vi "AB_820_850_Project_Build_Info.vi"(7 "action":T2, 8 "error in (no error)":errorcluster, 9 "buildType":T1, 10 "buildInfo in":T3, 11 "Object In":T4) -> (0 "error out":errorcluster, 2 "buildInfo out":T3, 3 "Object Out":T4)   [LabVIEW 2020]
uses:
  <resource>/Framework/Providers/API/ItemRef.ctl
  <vilib>/AppBuilder/RW_Project/AB_RW_Project_PropBag_Action.ctl
  <vilib>/AppBuilder/AB_BuildType.ctl
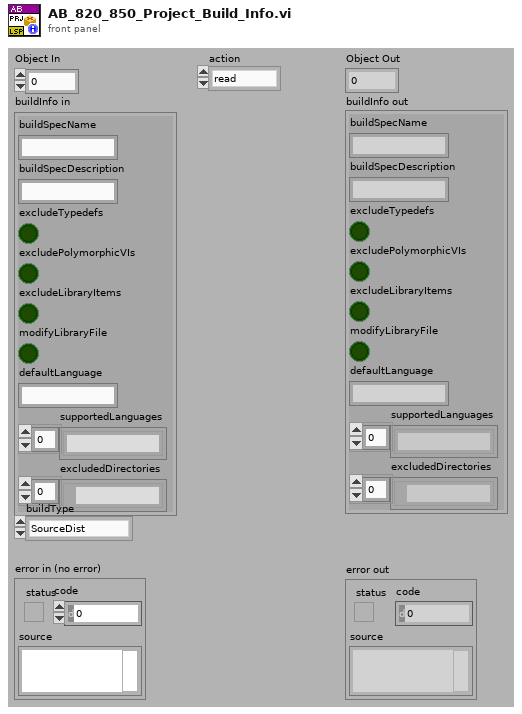
[diagram p1: front panel]
types:
  T1 = typedef "AB_BuildType.ctl" = enum16{"SourceDist", "EXE", "DLL", "RTExe"}
  T2 = typedef "AB_RW_Project_PropBag_Action.ctl" = enum16{"read", "write", "clear", "readPrevious", "writePrevious", "clearPrevious"}
  T3 = cluster{"buildSpecName":string, "buildSpecDescription":string, "excludeTypedefs":bool, "excludePolymorphicVIs":bool, "excludeLibraryItems":bool, "modifyLibraryFile":bool, "defaultLanguage":string, "supportedLanguages":string[], "excludedDirectories":path[]}
  T4 = typedef "ItemRef.ctl" = u64
  T5 = enum16{"<none>", "relativeToCommon", "relativeToAppDir"}
  T6 = typedef "AB_820_850_Relative_Path_Type.ctl" = enum16{"<none>", "relativeToCommon", "relativeToAppDir"}
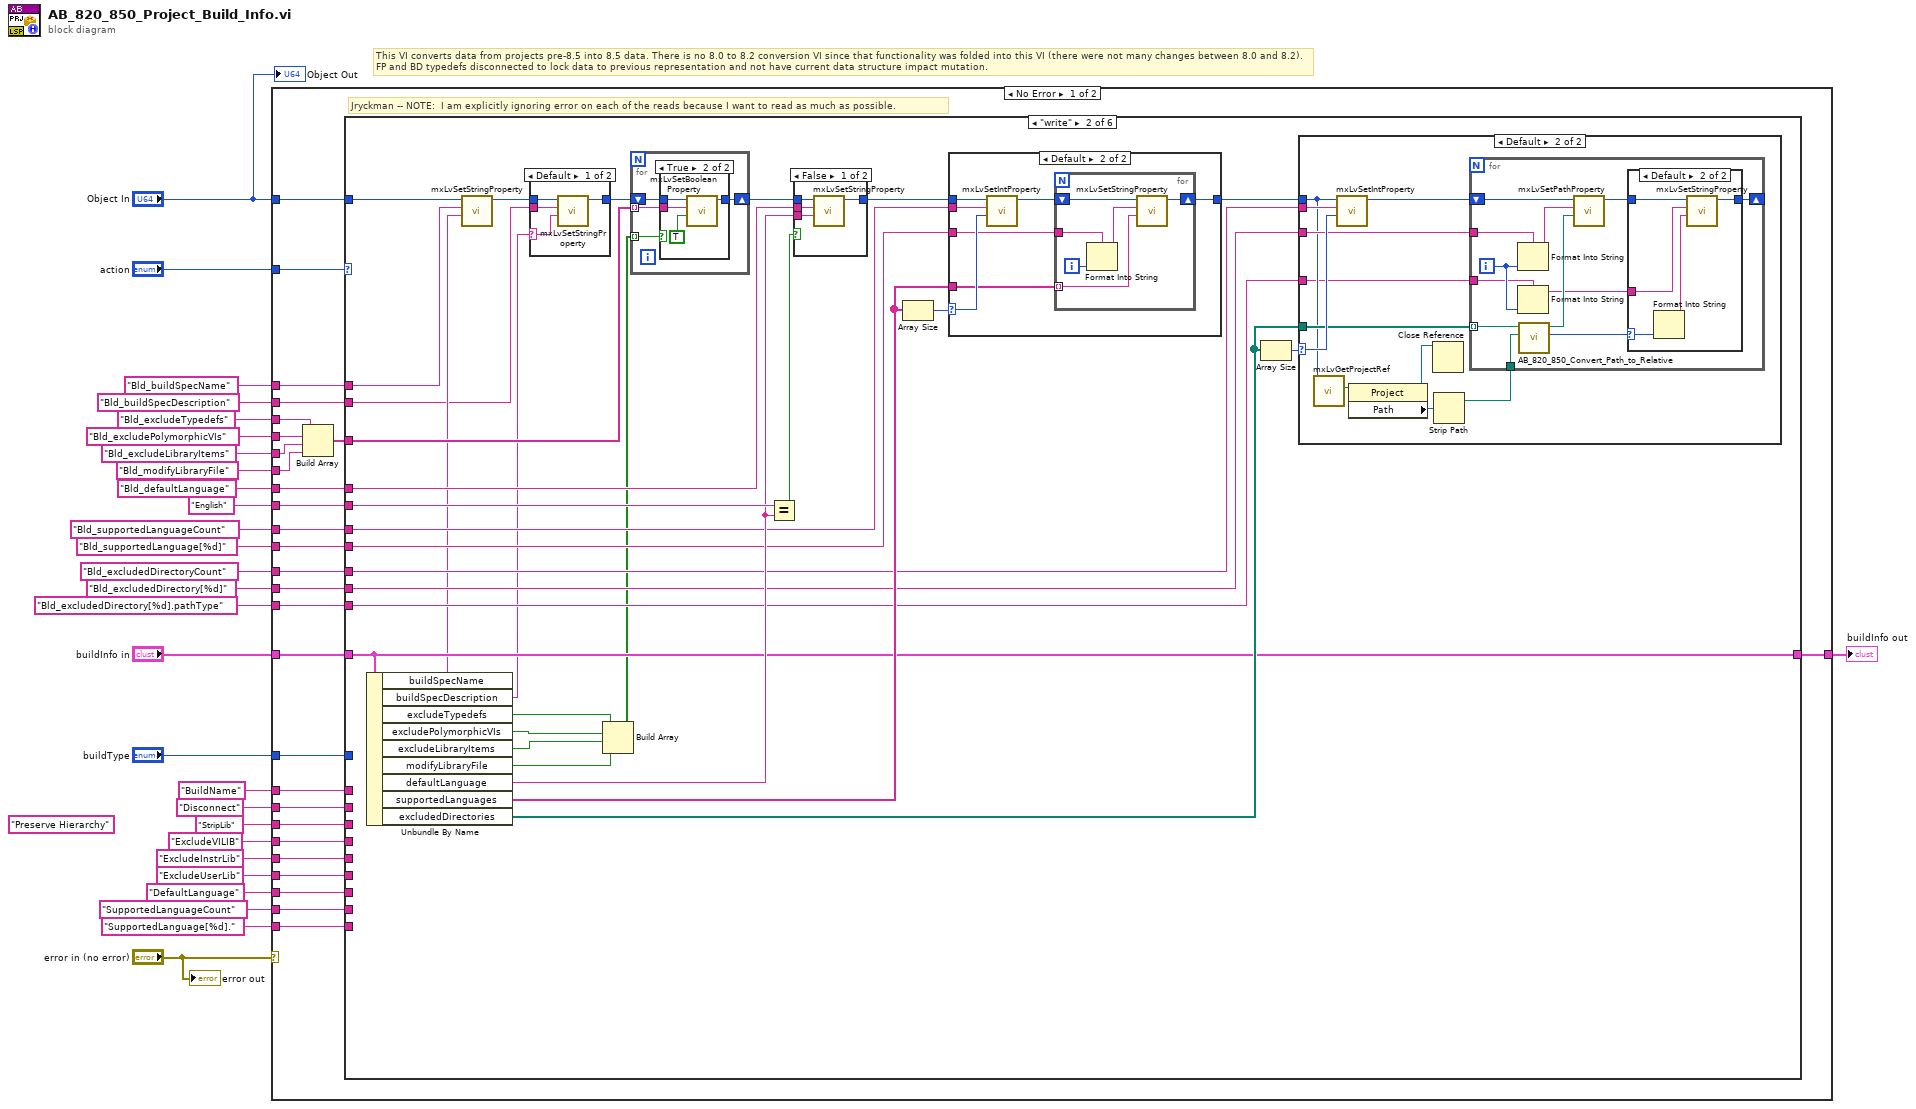
[diagram p0: block diagram]
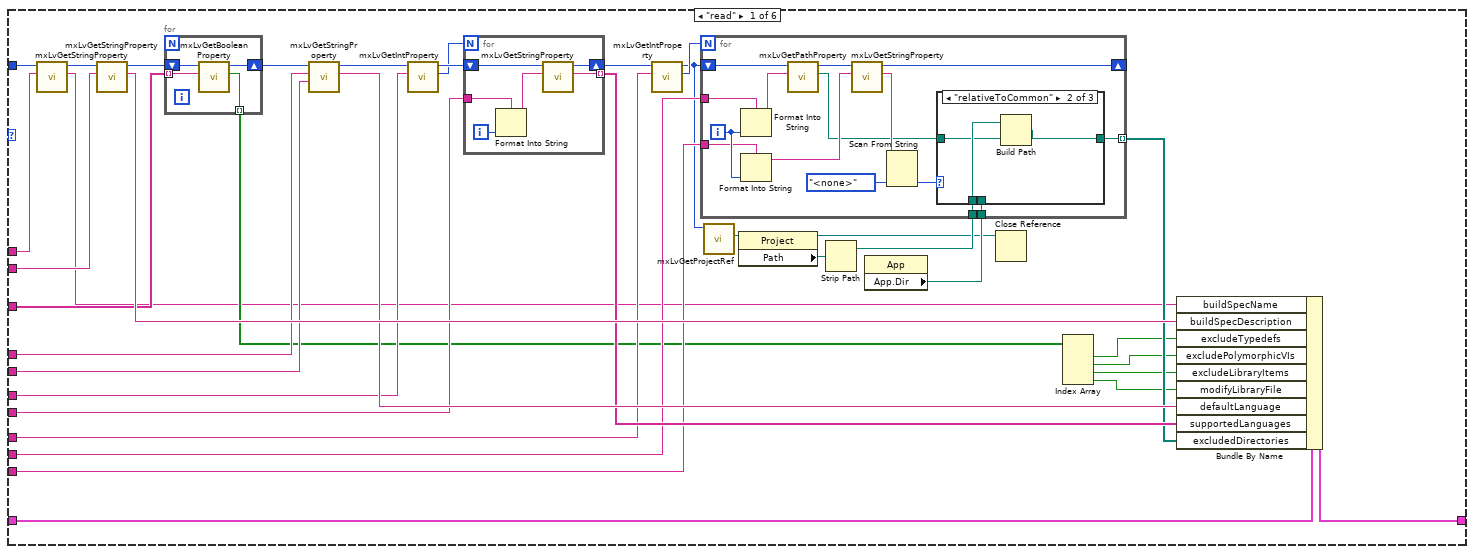
[diagram p2: hidden frame]
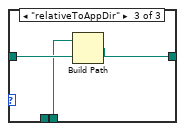
[diagram p4: hidden frame]
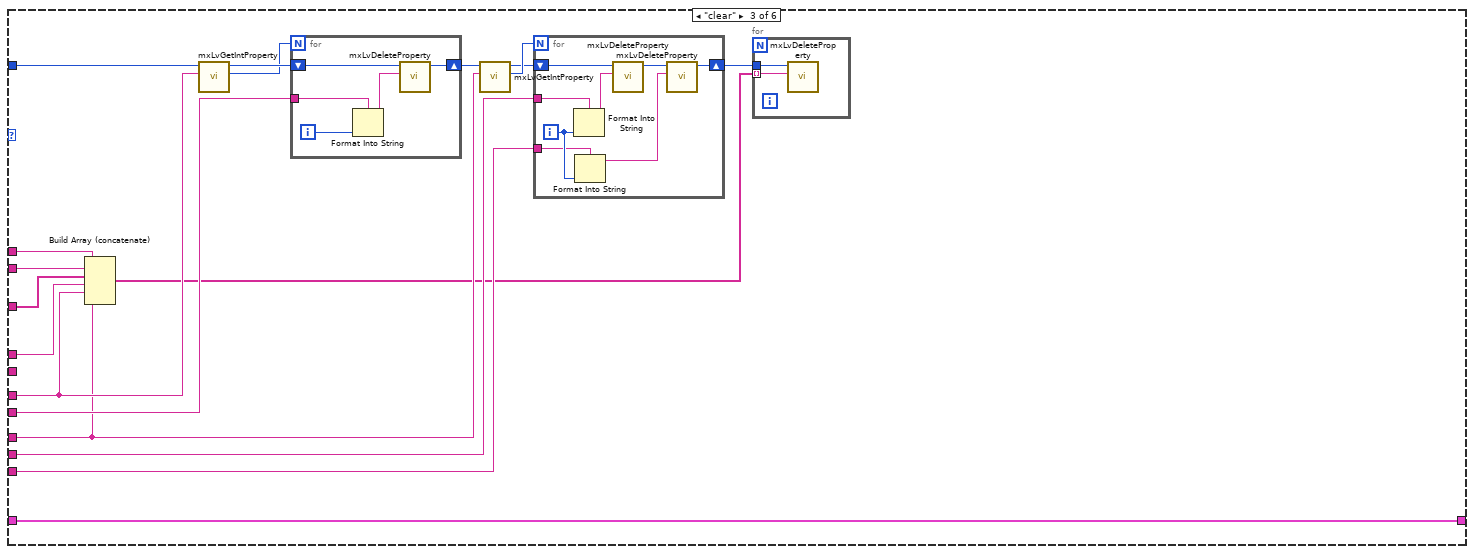
[diagram p11: hidden frame]
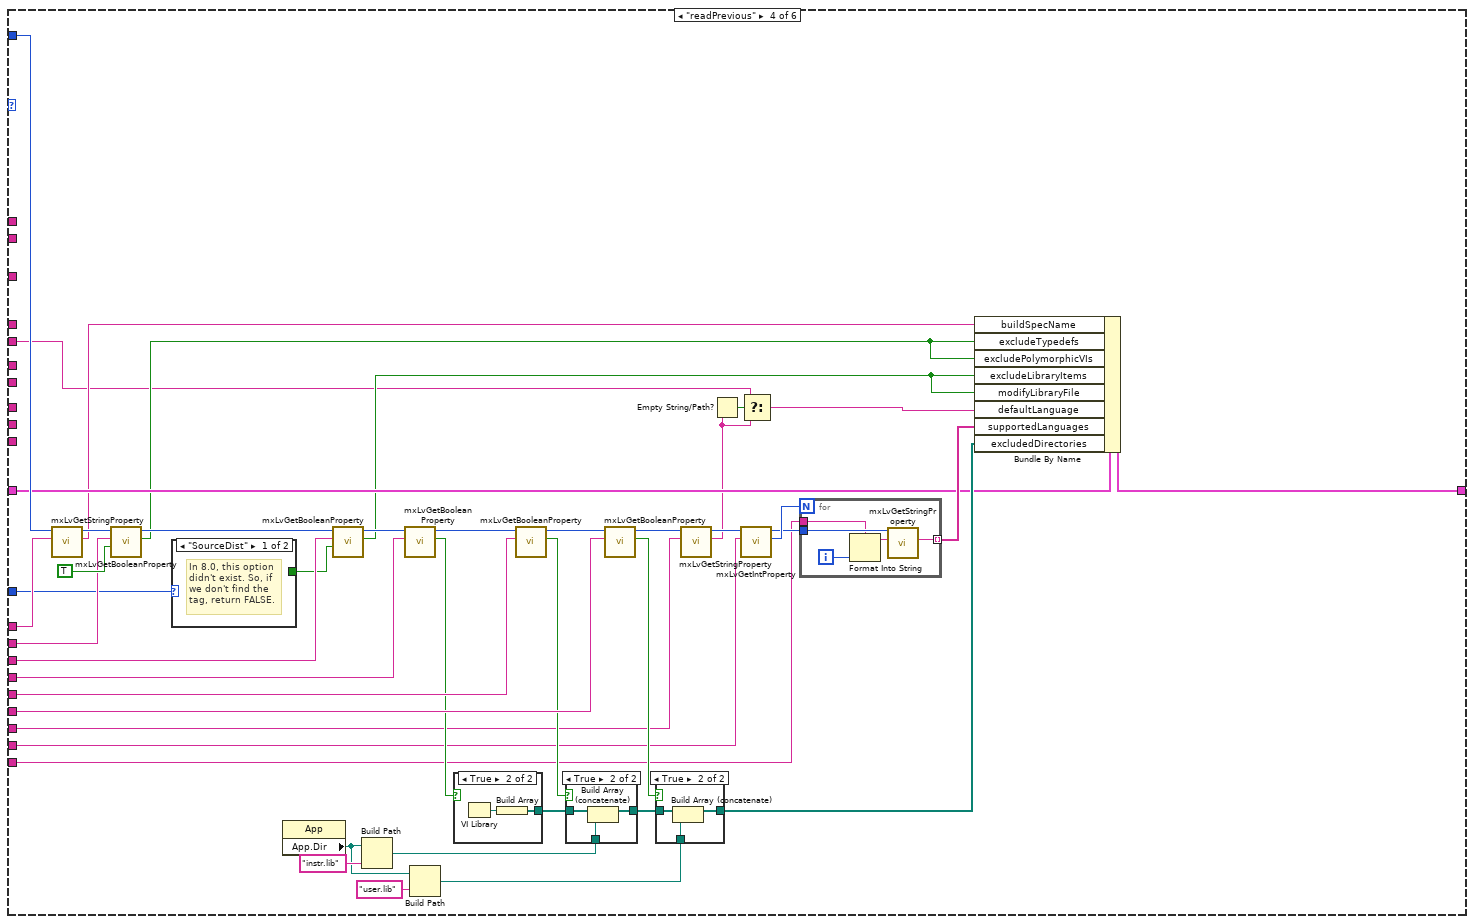
[diagram p12: hidden frame]
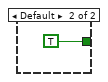
[diagram p13: hidden frame]
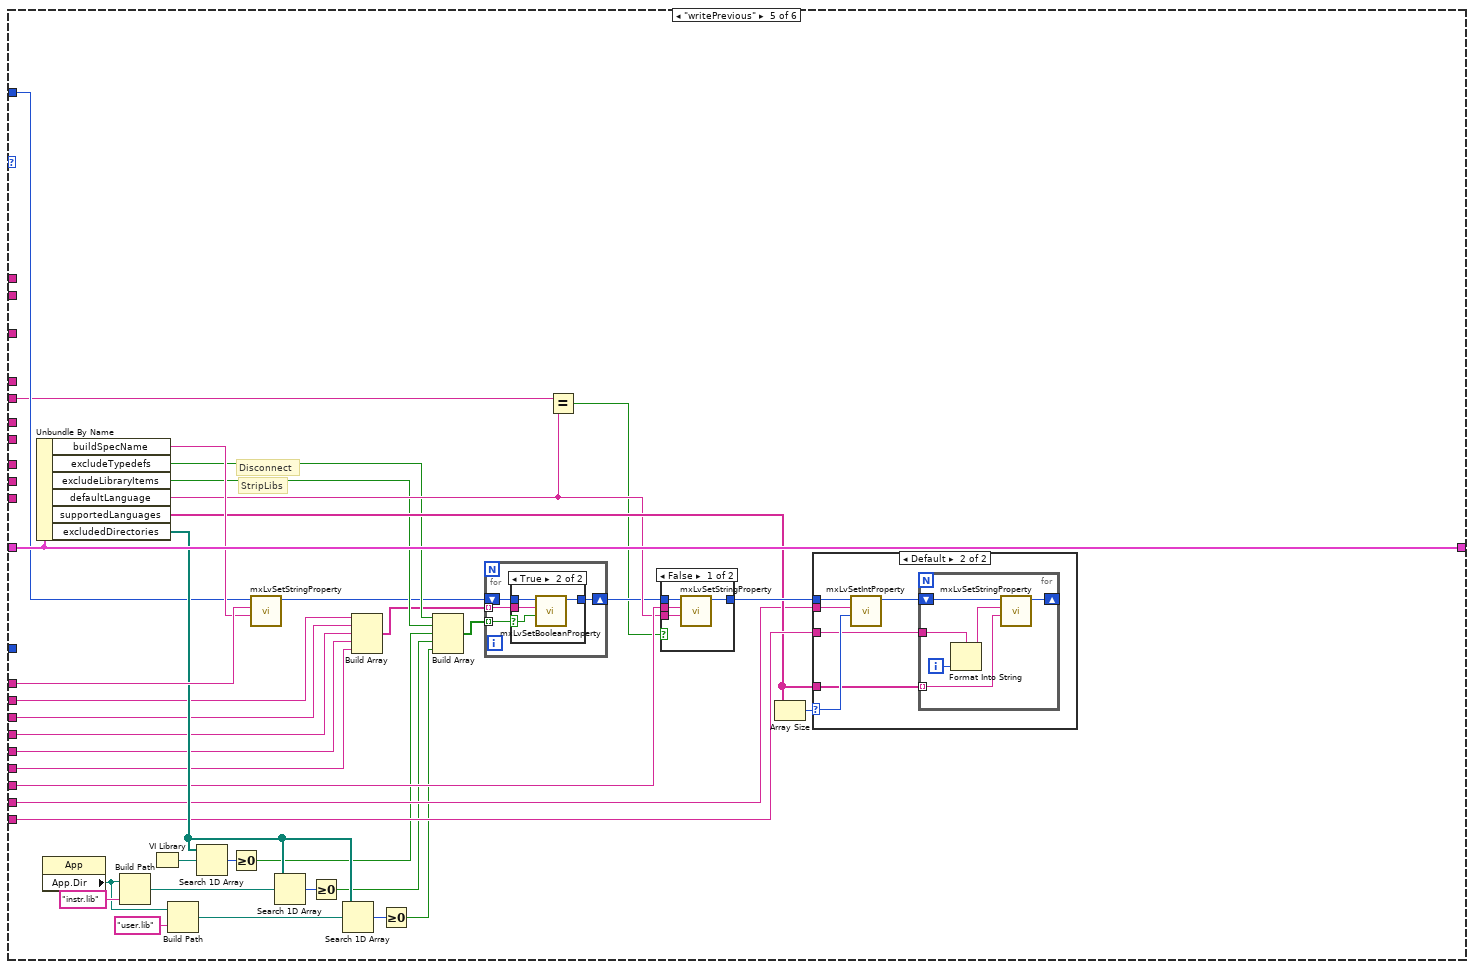
[diagram p17: hidden frame]
diagram:
  (unwired) "Preserve Hierarchy" ("Tag")
  # "This VI converts data from projects pre-8.5 into 8.5 data. There is no 8.0 to 8.2 conversion VI since that functionality was folded into this VI (there were not many changes between 8.0 and 8.2).\nFP and BD typedefs disconnected to lock data to previous representation and not have current data structure impact mutation."
  n1 = case shown="No Error" "error in (no error)" {
    tunnel: "Object In" -> [w56 _]
    tunnel: [w45 _] -> w26
    tunnel: "Bld_buildSpecDescription" ("Tag") -> [w55 _]
    tunnel: "Bld_excludeTypedefs" ("Tag") -> [w32 _]
    tunnel: "Bld_defaultLanguage" ("Tag") -> [w54 _]
    tunnel: "English" ("Tag") -> [w53 _]
    tunnel: "Bld_supportedLanguageCount" ("Tag") -> [w52 _]
    tunnel: "Bld_supportedLanguage[%d]" ("Tag") -> [w51 _]
    tunnel: "Bld_excludedDirectoryCount" ("Tag") -> [w50 _]
    tunnel: "Bld_excludedDirectory[%d]" ("Tag") -> [w49 _]
    tunnel: "Bld_excludedDirectory[%d].pathType" ("Tag") -> [w48 _]
    tunnel: "buildInfo in" -> [w47 _]
    tunnel: "action" -> [w46 _]
    tunnel: "BuildName" ("Tag") -> [w44 _]
    tunnel: "Disconnect" -> [w43 _]
    tunnel: "StripLib" -> [w42 _]
    tunnel: "ExcludeVILIB" -> [w41 _]
    tunnel: "ExcludeInstrLib" -> [w40 _]
    tunnel: "ExcludeUserLib" -> [w39 _]
    tunnel: "DefaultLanguage" ("Tag") -> [w38 _]
    tunnel: "SupportedLanguageCount" -> [w37 _]
    tunnel: "SupportedLanguage[%d]." ("string") -> [w36 _]
    tunnel: "Bld_excludePolymorphicVIs" ("Tag") -> [w35 _]
    tunnel: "Bld_excludeLibraryItems" ("Tag") -> [w34 _]
    tunnel: "Bld_modifyLibraryFile" ("Tag") -> [w33 _]
    tunnel: "Bld_buildSpecName" ("Tag") -> [w30 _]
    tunnel: "buildType" -> [w29 _]
    frame No Error {
      # "Jryckman -- NOTE:  I am explicitly ignoring error on each of the reads because I want to read as much as possible."
      n2 = Build Array(w32, w35, w34, w33) -> (w31:string[])
      n3 = case shown="\"write\"" w46 {
        tunnel: w56 -> [w61 w132 w233 w278 w333 w384]
        tunnel: w55 -> [w93 w127 w235 _ _ _]
        tunnel: w54 -> [w91 w154 w234 _ _ _]
        tunnel: w53 -> [w90 w153 _ w253 w330 _]
        tunnel: w52 -> [w87 w148 w232 _ _ _]
        tunnel: w51 -> [w84 w147 w229 _ _ _]
        tunnel: w50 -> [w81 w143 w225 _ _ _]
        tunnel: w49 -> [w79 w141 w224 _ _ _]
        tunnel: w48 -> [w78 w140 w223 _ _ _]
        tunnel: w47 -> [w70 w139 w220 w260 w342 w373]
        tunnel: [w71 w139 w220 w279 w342 w373] -> w45
        tunnel: w44 -> [_ _ _ w275 w343 w374]
        tunnel: w43 -> [_ _ _ w274 w322 w375]
        tunnel: w42 -> [_ _ _ w273 w321 w376]
        tunnel: w41 -> [_ _ _ w271 w320 w377]
        tunnel: w40 -> [_ _ _ w270 w319 w378]
        tunnel: w39 -> [_ _ _ w269 w318 w379]
        tunnel: w38 -> [_ _ _ w263 w326 w380]
        tunnel: w37 -> [_ _ _ w262 w327 w383]
        tunnel: w36 -> [_ _ _ w261 w329 w381]
        tunnel: w31 -> [w67 w133 w219 _ _ _]
        tunnel: w30 -> [w59 w130 w218 _ _ _]
        tunnel: w29 -> [_ _ _ w252 _ _]
        frame "read" {
          n4 = call <resource>:"mxLvGetStringProperty.vi"("Tag"=w59, "Item"=w61) -> ("Value"=w58:string, "Item"=w60:T4)  [unwired: 7 in, 1 out]
          n5 = call <resource>:"mxLvGetStringProperty.vi"("Tag"=w93, "Item"=w60) -> ("Value"=w92:string, "Item"=w69:T4)  [unwired: 7 in, 1 out]
          n6 = for {
            shift-right: [w97] -> w68
            shift-left: w69 -> [w95]
            tunnel: w67 -> [w96] mode=indexing
            tunnel: [w94] -> w66 mode=indexing
            n7 = call <resource>:"mxLvGetBooleanProperty.vi"("Tag"=w96, "Item"=w95) -> ("Value"=w94:bool, "Item"=w97:T4)  [unwired: 7 in, 1 out]
          }
          n8 = call <resource>:"mxLvGetStringProperty.vi"("Default Value (\"\")"=w90, "Tag"=w91, "Item"=w68) -> ("Value"=w89:string, "Item"=w88:T4)  [unwired: 6 in, 1 out]
          n9 = call <resource>:"mxLvGetIntProperty.vi"("Tag"=w87, "Item"=w88) -> ("Value"=w85:i32, "Item"=w86:T4)  [unwired: 7 in, 1 out]
          n10 = for {
            N: w85 -> [_]
            shift-right: [w122] -> w82
            shift-left: w86 -> [w123]
            tunnel: w84 -> [w124]
            tunnel: [w120] -> w83 mode=indexing
            i -> [w125]
            n11 = Format Into String(format string=w124, w125) -> (resulting string=w121:string)  [unwired: 2 in, 1 out]
            n12 = call <resource>:"mxLvGetStringProperty.vi"("Tag"=w121, "Item"=w123) -> ("Value"=w120:string, "Item"=w122:T4)  [unwired: 7 in, 1 out]
          }
          n13 = call <resource>:"mxLvGetIntProperty.vi"("Tag"=w81, "Item"=w82) -> ("Value"=w80:i32, "Item"=w75:T4)  [unwired: 7 in, 1 out]
          n14 = call <resource>:"mxLvGetProjectRef.vi"("Item"=w75) -> ("Project Refnum"=w77:refnum<vi>)  [unwired: 8 in, 2 out]
          n15 = property class="Project"(reference=w77) -> (reference out=w57:refnum<vi>, "Path"=w76:path)  [unwired: 1 in, 1 out]
          n16 = Strip Path(path=w76) -> (stripped path=w74:path)  [unwired: 1 out]
          n17 = property class="App"() -> ("App.Dir"=w72:path)  [unwired: 2 in, 2 out]
          n18 = for {
            N: w80 -> [_]
            shift-right: [w99] -> _
            shift-left: w75 -> [w109]
            tunnel: w79 -> [w112]
            tunnel: w78 -> [w110]
            tunnel: w74 -> [w102]
            tunnel: [w100] -> w73 mode=indexing
            tunnel: w72 -> [w98]
            i -> [w111]
            n19 = Format Into String(format string=w112, w111) -> (resulting string=w108:string)  [unwired: 2 in, 1 out]
            n20 = Format Into String(format string=w110, w111) -> (resulting string=w106:string)  [unwired: 2 in, 1 out]
            n21 = call <resource>:"mxLvGetPathProperty.vi"("Tag"=w108, "Item"=w109) -> ("Path"=w101:path, "Item"=w107:T4)  [unwired: 7 in, 1 out]
            n22 = call <resource>:"mxLvGetStringProperty.vi"("Tag"=w106, "Item"=w107) -> ("Value"=w105:string, "Item"=w99:T4)  [unwired: 7 in, 1 out]
            n23 = Scan From String(input string=w105, default 1=T5."<none>" ("relativeType")) -> (output 1=w103:T5)  [unwired: 3 in, 3 out]
            n24 = case shown="\"relativeToCommon\"" w103 {
              tunnel: w102 -> [_ w116 _]
              tunnel: w101 -> [w113 w115 w119]
              tunnel: [w113 w114 w118] -> w100
              tunnel: w98 -> [_ _ w117]
              frame "<none>" {
              }
              frame "relativeToCommon" {
                n25 = Build Path(base path=w116, name or relative path=w115) -> (appended path=w114:path)
              }
              frame "relativeToAppDir" {
                n26 = Build Path(base path=w117, name or relative path=w119) -> (appended path=w118:path)
              }
            }
          }
          n27 = Close Reference(reference=w57) -> ()  [unwired: 1 in, 1 out]
          n28 = Index Array(array=w66) -> (element #1=w65:bool, element #2=w64:bool, element #3=w63:bool, element #4=w62:bool)  [unwired: 4 in]
          n29 = Bundle By Name(cluster=w70, "buildSpecName"=w58, "buildSpecDescription"=w92, "excludeTypedefs"=w65, "excludePolymorphicVIs"=w64, "excludeLibraryItems"=w63, "modifyLibraryFile"=w62, "defaultLanguage"=w89, "supportedLanguages"=w83, "excludedDirectories"=w73) -> (w71:T3)
        }
        frame "write" {
          n30 = Unbundle By Name(w139) -> ("buildSpecName"=w131:string, "buildSpecDescription"=w126:string, "excludeTypedefs"=w138:bool, "excludePolymorphicVIs"=w137:bool, "excludeLibraryItems"=w136:bool, "modifyLibraryFile"=w135:bool, "defaultLanguage"=w152:string, "supportedLanguages"=w146:string[], "excludedDirectories"=w144:path[])
          n31 = call <resource>:"mxLvSetStringProperty.vi"("Value (\"\")"=w131, "Tag"=w130, "Item"=w132) -> ("Item"=w129:T4)  [unwired: 7 in, 1 out]
          n32 = case shown="Default" w126 {
            selector: w126 -> [w156 _]
            tunnel: w129 -> [w159 w160]
            tunnel: w127 -> [w158 _]
            tunnel: [w157 w160] -> w128
            frame Default {
              n33 = call <resource>:"mxLvSetStringProperty.vi"("Value (\"\")"=w156, "Tag"=w158, "Item"=w159) -> ("Item"=w157:T4)  [unwired: 7 in, 1 out]
            }
            frame "" {
            }
          }
          n34 = Build Array(w138, w137, w136, w135) -> (w134:bool[])
          n35 = for {
            shift-right: [w163] -> w155
            shift-left: w128 -> [w164]
            tunnel: w134 -> [w162] mode=indexing
            tunnel: w133 -> [w161] mode=indexing
            n36 = case shown="True" w162 {
              tunnel: w164 -> [w165 w169]
              tunnel: [w165 w168] -> w163
              tunnel: w161 -> [_ w167]
              frame False {
              }
              frame True {
                n37 = call <resource>:"mxLvSetBooleanProperty.vi"("Value (F)"=TRUE, "Tag"=w167, "Item"=w169) -> ("Item"=w168:T4)  [unwired: 7 in, 1 out]
              }
            }
          }
          n38 = Equal?(x=w153, y=w152) -> (x = y?=w151:bool)
          n39 = case shown="False" w151 {
            tunnel: w155 -> [w216 w217]
            tunnel: w154 -> [w215 _]
            tunnel: w152 -> [w214 _]
            tunnel: [w213 w217] -> w149
            frame False {
              n40 = call <resource>:"mxLvSetStringProperty.vi"("Value (\"\")"=w214, "Tag"=w215, "Item"=w216) -> ("Item"=w213:T4)  [unwired: 7 in, 1 out]
            }
            frame True {
            }
          }
          n41 = Array Size(array=w146) -> (size(s)=w150:i32)
          n42 = case shown="Default" w150 {
            selector: w150 -> [_ w204]
            tunnel: w149 -> [w199 w206]
            tunnel: w148 -> [_ w205]
            tunnel: w147 -> [_ w202]
            tunnel: w146 -> [_ w201]
            tunnel: [w199 w200] -> w142
            frame 0 {
            }
            frame Default {
              n43 = call <resource>:"mxLvSetIntProperty.vi"("Value (0)"=w204, "Tag"=w205, "Item"=w206) -> ("Item"=w203:T4)  [unwired: 7 in, 1 out]
              n44 = for {
                shift-right: [w211] -> w200
                shift-left: w203 -> [w212]
                tunnel: w202 -> [w209]
                tunnel: w201 -> [w207] mode=indexing
                i -> [w210]
                n45 = Format Into String(format string=w209, w210) -> (resulting string=w208:string)  [unwired: 2 in, 1 out]
                n46 = call <resource>:"mxLvSetStringProperty.vi"("Value (\"\")"=w207, "Tag"=w208, "Item"=w212) -> ("Item"=w211:T4)  [unwired: 7 in, 1 out]
              }
            }
          }
          n47 = Array Size(array=w144) -> (size(s)=w145:i32)
          n48 = case shown="Default" w145 {
            selector: w145 -> [_ w179]
            tunnel: w142 -> [_ w175]
            tunnel: w143 -> [_ w180]
            tunnel: w141 -> [_ w177]
            tunnel: w144 -> [_ w176]
            tunnel: w140 -> [_ w172]
            frame 0 {
            }
            frame Default {
              n49 = call <resource>:"mxLvGetProjectRef.vi"("Item"=w175) -> ("Project Refnum"=w174:refnum<vi>)  [unwired: 8 in, 2 out]
              n50 = call <resource>:"mxLvSetIntProperty.vi"("Value (0)"=w179, "Tag"=w180, "Item"=w175) -> ("Item"=w178:T4)  [unwired: 7 in, 1 out]
              n51 = property class="Project"(reference=w174) -> (reference out=w170:refnum<vi>, "Path"=w173:path)  [unwired: 1 in, 1 out]
              n52 = Close Reference(reference=w170) -> ()  [unwired: 1 in, 1 out]
              n53 = Strip Path(path=w173) -> (stripped path=w171:path)  [unwired: 1 out]
              n54 = for {
                shift-right: [w192] -> _
                shift-left: w178 -> [w188]
                tunnel: w177 -> [w191]
                tunnel: w176 -> [w190] mode=indexing
                tunnel: w171 -> [w182]
                tunnel: w172 -> [w181]
                i -> [w186]
                n55 = Format Into String(format string=w191, w186) -> (resulting string=w189:string)  [unwired: 2 in, 1 out]
                n56 = Format Into String(format string=w181, w186) -> (resulting string=w184:string)  [unwired: 2 in, 1 out]
                n57 = call <vilib>:"AB_820_850_Convert_Path_to_Relative.vi"("commonPath"=w182, "absolutePath"=w190) -> ("relativeType"=w183:T6, "newPath"=w185:path)  [unwired: 7 in, 1 out]
                n58 = call <resource>:"mxLvSetPathProperty.vi"("Path"=w185, "Tag"=w189, "Item"=w188) -> ("Item"=w187:T4)  [unwired: 7 in, 1 out]
                n59 = case shown="Default" w183 {
                  selector: w183 -> [_ w194]
                  tunnel: [w193 w198] -> w192
                  tunnel: w187 -> [w193 w197]
                  tunnel: w184 -> [_ w195]
                  frame "<none>" {
                  }
                  frame Default {
                    n60 = Format Into String(w194) -> (resulting string=w196:string)  [unwired: 3 in, 1 out]
                    n61 = call <resource>:"mxLvSetStringProperty.vi"("Value (\"\")"=w196, "Tag"=w195, "Item"=w197) -> ("Item"=w198:T4)  [unwired: 7 in, 1 out]
                  }
                }
              }
            }
          }
        }
        frame "clear" {
          n62 = Build Array (concatenate)(w218, w235, w219, w234, w232, w225) -> (w221:string[])
          n63 = call <resource>:"mxLvGetIntProperty.vi"("Tag"=w232, "Item"=w233) -> ("Value"=w230:i32, "Item"=w231:T4)  [unwired: 7 in, 1 out]
          n64 = for {
            N: w230 -> [_]
            shift-right: [w247] -> w226
            shift-left: w231 -> [w248]
            tunnel: w229 -> [w249]
            i -> [w250]
            n65 = Format Into String(format string=w249, w250) -> (resulting string=w246:string)  [unwired: 2 in, 1 out]
            n66 = call <resource>:"mxLvDeleteProperty.vi"("Tag"=w246, "Item"=w248) -> ("Item"=w247:T4)  [unwired: 8 in, 1 out]
          }
          n67 = call <resource>:"mxLvGetIntProperty.vi"("Tag"=w225, "Item"=w226) -> ("Value"=w228:i32, "Item"=w227:T4)  [unwired: 7 in, 1 out]
          n68 = for {
            N: w228 -> [_]
            shift-right: [w241] -> w222
            shift-left: w227 -> [w244]
            tunnel: w224 -> [w245]
            tunnel: w223 -> [w239]
            i -> [w240]
            n69 = Format Into String(format string=w245, w240) -> (resulting string=w243:string)  [unwired: 2 in, 1 out]
            n70 = Format Into String(format string=w239, w240) -> (resulting string=w238:string)  [unwired: 2 in, 1 out]
            n71 = call <resource>:"mxLvDeleteProperty.vi"("Tag"=w243, "Item"=w244) -> ("Item"=w242:T4)  [unwired: 8 in, 1 out]
            n72 = call <resource>:"mxLvDeleteProperty.vi"("Tag"=w238, "Item"=w242) -> ("Item"=w241:T4)  [unwired: 8 in, 1 out]
          }
          n73 = for {
            tunnel: w222 -> [w237]
            tunnel: w221 -> [w236] mode=indexing
            n74 = call <resource>:"mxLvDeleteProperty.vi"("Tag"=w236, "Item"=w237) -> ()  [unwired: 8 in, 2 out]
          }
        }
        frame "readPrevious" {
          n75 = call <resource>:"mxLvGetStringProperty.vi"("Tag"=w275, "Item"=w278) -> ("Value"=w259:string, "Item"=w277:T4)  [unwired: 7 in, 1 out]
          n76 = call <resource>:"mxLvGetBooleanProperty.vi"("Default Value (F)"=TRUE, "Tag"=w274, "Item"=w277) -> ("Value"=w258:bool, "Item"=w291:T4)  [unwired: 6 in, 1 out]
          n77 = case shown="\"SourceDist\"" w252 {
            tunnel: [_ TRUE ("Default Value (F)")] -> w251
            frame "SourceDist" {
              # "In 8.0, this option didn't exist. So, if we don't find the tag, return FALSE."
            }
            frame Default {
            }
          }
          n78 = property class="App"() -> ("App.Dir"=w282:path)  [unwired: 2 in, 2 out]
          n79 = call <resource>:"mxLvGetBooleanProperty.vi"("Default Value (F)"=w251, "Tag"=w273, "Item"=w291) -> ("Value"=w257:bool, "Item"=w272:T4)  [unwired: 6 in, 1 out]
          n80 = Build Path(base path=w282, name or relative path="instr.lib") -> (appended path=w283:path)
          n81 = call <resource>:"mxLvGetBooleanProperty.vi"("Tag"=w271, "Item"=w272) -> ("Value"=w268:bool, "Item"=w289:T4)  [unwired: 7 in, 1 out]
          n82 = Build Path(base path=w282, name or relative path="user.lib") -> (appended path=w280:path)
          n83 = case shown="True" w268 {
            tunnel: [_ w303] -> w287
            frame False {
            }
            frame True {
              n84 = VI Library() -> (path=w304:path)
              n85 = Build Array(w304) -> (w303:path[])
            }
          }
          n86 = call <resource>:"mxLvGetBooleanProperty.vi"("Tag"=w270, "Item"=w289) -> ("Value"=w267:bool, "Item"=w288:T4)  [unwired: 7 in, 1 out]
          n87 = case shown="True" w267 {
            tunnel: [w299 w302] -> w286
            tunnel: w287 -> [w299 w301]
            tunnel: w283 -> [_ w300]
            frame False {
            }
            frame True {
              n88 = Build Array (concatenate)(w301, w300) -> (w302:path[])
            }
          }
          n89 = call <resource>:"mxLvGetBooleanProperty.vi"("Tag"=w269, "Item"=w288) -> ("Value"=w266:bool, "Item"=w264:T4)  [unwired: 7 in, 1 out]
          n90 = case shown="True" w266 {
            tunnel: [w295 w298] -> w285
            tunnel: w286 -> [w295 w297]
            tunnel: w280 -> [_ w296]
            frame False {
            }
            frame True {
              n91 = Build Array (concatenate)(w297, w296) -> (w298:path[])
            }
          }
          n92 = call <resource>:"mxLvGetStringProperty.vi"("Tag"=w263, "Item"=w264) -> ("Value"=w255:string, "Item"=w265:T4)  [unwired: 7 in, 1 out]
          n93 = Empty String/Path?(string/path=w255) -> (empty?=w256:bool)
          n94 = call <resource>:"mxLvGetIntProperty.vi"("Tag"=w262, "Item"=w265) -> ("Value"=w293:i32, "Item"=w292:T4)  [unwired: 7 in, 1 out]
          n95 = Select(t=w253, s=w256, f=w255) -> (s? t:f=w254:string)
          n96 = for {
            N: w293 -> [_]
            tunnel: [w308] -> w290 mode=indexing
            tunnel: w292 -> [w309]
            tunnel: w261 -> [w305]
            i -> [w307]
            n97 = Format Into String(format string=w305, w307) -> (resulting string=w306:string)  [unwired: 2 in, 1 out]
            n98 = call <resource>:"mxLvGetStringProperty.vi"("Tag"=w306, "Item"=w309) -> ("Value"=w308:string)  [unwired: 7 in, 2 out]
          }
          n99 = Bundle By Name(cluster=w260, "buildSpecName"=w259, "excludeTypedefs"=w258, "excludePolymorphicVIs"=w258, "excludeLibraryItems"=w257, "modifyLibraryFile"=w257, "defaultLanguage"=w254, "supportedLanguages"=w290, "excludedDirectories"=w285) -> (w279:T3)
        }
        frame "writePrevious" {
          # "Disconnect"
          # "StripLibs"
          n100 = Unbundle By Name(w342) -> ("buildSpecName"=w341:string, "excludeTypedefs"=w317:bool, "excludeLibraryItems"=w316:bool, "defaultLanguage"=w325:string, "supportedLanguages"=w328:string[], "excludedDirectories"=w340:path[])
          n101 = property class="App"() -> ("App.Dir"=w345:path)  [unwired: 2 in, 2 out]
          n102 = Build Path(base path=w345, name or relative path="instr.lib") -> (appended path=w335:path)
          n103 = VI Library() -> (path=w336:path)
          n104 = Build Path(base path=w345, name or relative path="user.lib") -> (appended path=w334:path)
          n105 = Search 1D Array(1D array=w340, element=w336) -> (index of element=w339:i32)  [unwired: 1 in]
          n106 = Greater Or Equal To 0?(x=w339) -> (x >= 0?=w315:bool)
          n107 = call <resource>:"mxLvSetStringProperty.vi"("Value (\"\")"=w341, "Tag"=w343, "Item"=w333) -> ("Item"=w312:T4)  [unwired: 7 in, 1 out]
          n108 = Search 1D Array(1D array=w340, element=w335) -> (index of element=w338:i32)  [unwired: 1 in]
          n109 = Greater Or Equal To 0?(x=w338) -> (x >= 0?=w314:bool)
          n110 = Search 1D Array(1D array=w340, element=w334) -> (index of element=w337:i32)  [unwired: 1 in]
          n111 = Build Array(w322, w321, w320, w319, w318) -> (w311:string[])
          n112 = Greater Or Equal To 0?(x=w337) -> (x >= 0?=w313:bool)
          n113 = Build Array(w317, w316, w315, w314, w313) -> (w310:bool[])
          n114 = for {
            shift-right: [w350] -> w324
            shift-left: w312 -> [w349]
            tunnel: w311 -> [w348] mode=indexing
            tunnel: w310 -> [w347] mode=indexing
            n115 = case shown="True" w347 {
              selector: w347 -> [_ w352]
              tunnel: [w351 w355] -> w350
              tunnel: w349 -> [w351 w354]
              tunnel: w348 -> [_ w353]
              frame False {
              }
              frame True {
                n116 = call <resource>:"mxLvSetBooleanProperty.vi"("Value (F)"=w352, "Tag"=w353, "Item"=w354) -> ("Item"=w355:T4)  [unwired: 7 in, 1 out]
              }
            }
          }
          n117 = Equal?(x=w330, y=w325) -> (x = y?=w323:bool)
          n118 = case shown="False" w323 {
            tunnel: w324 -> [w371 w372]
            tunnel: w326 -> [w370 _]
            tunnel: w325 -> [w369 _]
            tunnel: [w368 w372] -> w331
            frame False {
              n119 = call <resource>:"mxLvSetStringProperty.vi"("Value (\"\")"=w369, "Tag"=w370, "Item"=w371) -> ("Item"=w368:T4)  [unwired: 7 in, 1 out]
            }
            frame True {
            }
          }
          n120 = Array Size(array=w328) -> (size(s)=w332:i32)
          n121 = case shown="Default" w332 {
            selector: w332 -> [_ w359]
            tunnel: w331 -> [_ w361]
            tunnel: w327 -> [_ w360]
            tunnel: w329 -> [_ w357]
            tunnel: w328 -> [_ w356]
            frame 0 {
            }
            frame Default {
              n122 = call <resource>:"mxLvSetIntProperty.vi"("Value (0)"=w359, "Tag"=w360, "Item"=w361) -> ("Item"=w358:T4)  [unwired: 7 in, 1 out]
              n123 = for {
                shift-right: [w366] -> _
                shift-left: w358 -> [w367]
                tunnel: w357 -> [w364]
                tunnel: w356 -> [w362] mode=indexing
                i -> [w365]
                n124 = Format Into String(format string=w364, w365) -> (resulting string=w363:string)  [unwired: 2 in, 1 out]
                n125 = call <resource>:"mxLvSetStringProperty.vi"("Value (\"\")"=w362, "Tag"=w363, "Item"=w367) -> ("Item"=w366:T4)  [unwired: 7 in, 1 out]
              }
            }
          }
        }
        frame "clearPrevious" {
          n126 = Build Array(w374, w375, w376, w377, w378, w379, w380, w383) -> (w385:string[])
          n127 = call <resource>:"mxLvGetIntProperty.vi"("Tag"=w383, "Item"=w384) -> ("Value"=w386:i32, "Item"=w387:T4)  [unwired: 7 in, 1 out]
          n128 = for {
            N: w386 -> [_]
            shift-right: [w391] -> w382
            shift-left: w387 -> [w392]
            tunnel: w381 -> [w393]
            i -> [w394]
            n129 = Format Into String(format string=w393, w394) -> (resulting string=w390:string)  [unwired: 2 in, 1 out]
            n130 = call <resource>:"mxLvDeleteProperty.vi"("Tag"=w390, "Item"=w392) -> ("Item"=w391:T4)  [unwired: 8 in, 1 out]
          }
          n131 = for {
            tunnel: w382 -> [w389]
            tunnel: w385 -> [w388] mode=indexing
            n132 = call <resource>:"mxLvDeleteProperty.vi"("Tag"=w388, "Item"=w389) -> ()  [unwired: 8 in, 2 out]
          }
        }
      }
    }
    frame Error {
    }
  }
  "buildInfo out" <- w26
  "Object Out" <- "Object In"
  "error out" <- "error in (no error)"
